vi "Find Missing Hardware Identifiers.vi"(8 "error in (no error)":errorcluster, 11 "Routing and Faulting Custom Device Ref in":T2 format="%.0x") -> (0 "error out":errorcluster, 1 "Identifier Errors":errorcluster[](array[cluster]), 2 "Missing Identifiers":T1[](array[typedef]), 3 "Routing and Faulting Custom Device Ref out":T2 format="%.0x")   [LabVIEW 2017, in "Routing and Faulting Scripting.lvlib"]
uses:
  Routing and Faulting Scripting.lvlib
  <vilib>/NI Veristand/Custom Device API/Custom Device Item Ref.ctl
  Identifier Path Pair.ctl
  NationalInstruments.VeriStand.SystemStorage
  Constants/Scripting Constants.vi
  <vilib>/NI Veristand/Custom Device API/Custom Device API.lvlib
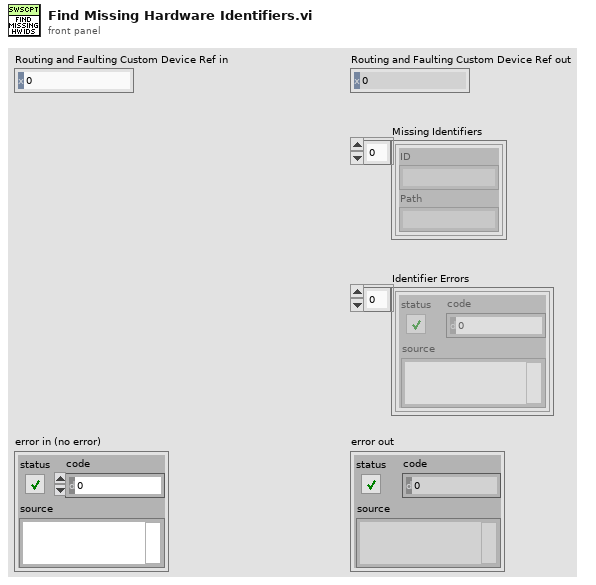
[diagram p1: front panel]
types:
  T1 = typedef "Routing and Faulting Scripting.lvlib/Identifier Path Pair.ctl" = cluster{"ID":string, "Path":string}
  T2 = typedef "Custom Device API.lvlib/Custom Device Item Ref.ctl" = u64
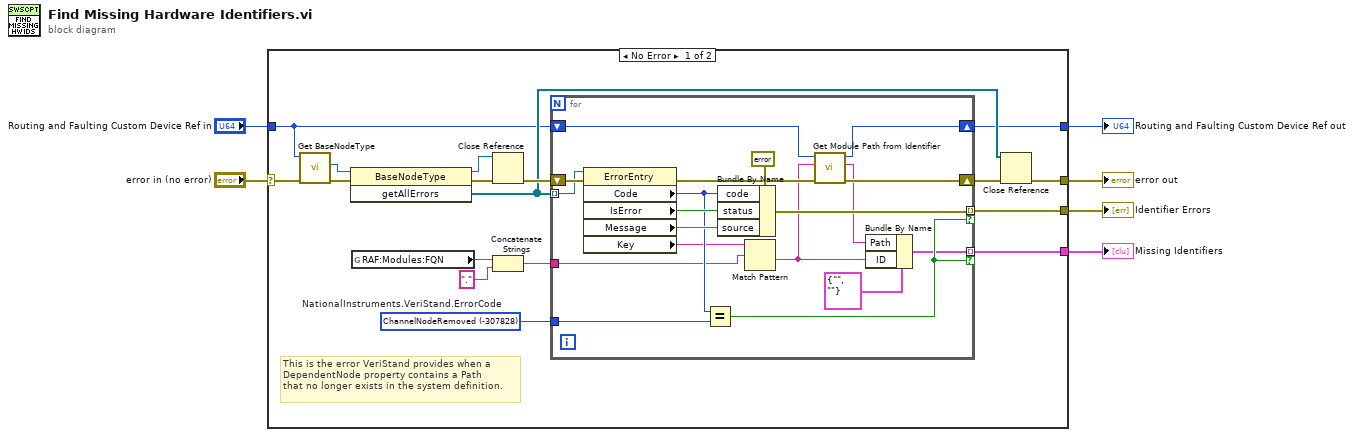
[diagram p0: block diagram]
diagram:
  n1 = case shown="No Error" "error in (no error)" {
    selector: "error in (no error)" -> [w15 w43]
    tunnel: "Routing and Faulting Custom Device Ref in" -> [w8 w44]
    tunnel: [w7 w44] -> w4
    tunnel: [w14 w43] -> w3
    tunnel: [w13 _] -> w2
    tunnel: [w12 _] -> w1
    frame No Error {
      w17 = -307828 items=["Success"=0, "NoProjectOpen"=-307992, "SequenceCompileError"=-307988, "SessionAlreadyDeployed"=-307984, "SessionNotDeployed"=-307982, "SequenceNotFoundInSession"=-307981, "StimulusProfileSessionLocked"=-307980, "EmptyNodeName"=-307930, "NodeAlreadyExistsByName"=-307926, "NumberOfCoefficientsOutOfRange"=-307884, "DownloadFileError"=-307872, "IncorrectLogFileName"=-307871, "LogTriggerConditionSyntaxError"=-307868, "DuplicateLogSessionName"=-307867, "LogSessionNotFound"=-307865, "ChannelLengthMismatch"=-307830, "NodeNotFoundDuringCompile"=-307829, "ChannelNodeRemoved"=-307828, "NotAChannel"=-307825, "NotAWaveform"=-307824, "STIFileError"=-307784, "DependenciesCycle"=-307783, "ChannelNotFoundInLogFile"=-307782, "ChannelGroupNotFoundInLogFile"=-307781, "GatewayNotOnLocalhost"=-307780, "NotEnoughDynamicDataSharingSpace"=-307738, "TargetMissingDataSharingDevice"=-307737, "ChannelMappingsSizeMismatch"=-307728, "DuplicateChannelAliasMappings"=-307711, "NotAnInlineCustomDevice"=-307710, "IncompatibleModel"=-307703, "ModelDimensionMismatch"=-307702, "SLSCChassisLoadFailed"=-307691, "TargetDisabled"=-307689, "MismatchedLengths"=-307687, "TargetInvalid"=-307686, "ParameterNotFound"=-307685, "ServerPortAlreadyInUse"=-307684, "TargetDisconnected"=-307682, "ServiceConfigurationFile"=-307681, "ModelParameterFileParseError"=-307680, "NoActionRequired"=-307677, "InputParameterInvalid"=-307676, "HostRunningDifferentSystemDefinition"=-307671, "ChannelNotScalable"=-307668, "ChannelCannotBeFaulted"=-307666, "ChannelNotWritable"=-307665, "ChannelNotReadable"=-307664, "Timeout"=-307663, "NodeNotFound"=-307662, "SystemDefinitionDeploymentFailure"=-307661, "SystemDefinitionDeploymentTimeout"=-307660, "EmptyPassword"=-307659, "SystemDefinitionAlreadyActive"=-307658, "InvalidConfigurationPassword"=-307657, "NoSystemDefinitionLoaded"=-307656, "ComponentNotAvailable"=-307655, "NotDeployed"=-307654, "InvalidFile"=-307653, "FailedServerConnection"=-307652, "FunctionNotSupported"=-307651, "UnexpectedError"=-307650, "UnmappedAlias"=-307617, "InvalidStreamConditionForDataType"=-307554, "WaveformDataTypeMismatch"=-307553, "InvalidDaqPluginFile"=-307526, "FileVersionUnsupported"=-307525]  # NationalInstruments.VeriStand.ErrorCode
      # "This is the error VeriStand provides when a\nDependentNode property contains a Path\nthat no longer exists in the system definition."
      n2 = call "Get BaseNodeType.vi"("error in (no error)"=w15, "Item Ref in"=w8) -> ("error out"=w23:errorcluster, "BaseNodeType"=w22:refnum<k24>)  [unwired: 7 in, 1 out]
      n3 = invoke class="BaseNodeType" method="getAllErrors"(reference=w22, error in=w23) -> (reference out=w20:refnum<k24>, error out=w21:errorcluster, "getAllErrors"=w16:refnum<k24>[])  [unwired: 1 in]
      n4 = global read "Scripting Constants.vi" "RAF:Modules:FQN"() -> (w11:string)
      n5 = Close Reference(reference=w20, error in (no error)=w21) -> (error out=w19:errorcluster)
      n6 = Concatenate Strings(w11, "." ("string")) -> (w9:string)
      n7 = for {
        shift-right: [w28] -> w18
        shift-left: w19 -> [w42]
        tunnel: w16 -> [w41] mode=indexing
        tunnel: [w37] -> w13 mode=indexing if=w34
        tunnel: w17 -> [w36]
        tunnel: [w24] -> w12 mode=indexing if=w34
        tunnel: w9 -> [w32]
        shift-right: [w29] -> w7
        shift-left: w8 -> [w30]
        n8 = property class="ErrorEntry"(reference=w41, error in=w42) -> (error out=w31:errorcluster, "Code"=w35:i32, "IsError"=w39:bool, "Message"=w38:string, "Key"=w33:string)  [unwired: 1 out]
        n9 = Equal?(x=w35, y=w36) -> (x = y?=w34:bool)
        n10 = Bundle By Name(cluster=errorcluster {"status"=FALSE, "code"=0, "source"=""} ("error out"), "code"=w35, "status"=w39, "source"=w38) -> (w37:errorcluster)
        n11 = Match Pattern(string=w33, regular expression=w32) -> (after substring=w26:string)  [unwired: 1 in, 3 out]
        n12 = call "Get Module Path from Identifier.vi"("error in (no error)"=w31, "Module identifier"=w26, "Routing and Faulting Ref in"=w30) -> ("error out"=w28:errorcluster, "Module path"=w25:string, "Routing and Faulting Ref out"=w29:T2)  [unwired: 6 in]
        n13 = Bundle By Name(cluster=T1 {"ID"="", "Path"=""}, "Path"=w25, "ID"=w26) -> (w24:T1)
      }
      n14 = Close Reference(reference=w16, error in (no error)=w18) -> (error out=w14:errorcluster)
    }
    frame Error {
    }
  }
  "Routing and Faulting Custom Device Ref out" <- w4
  "error out" <- w3
  "Identifier Errors" <- w2
  "Missing Identifiers" <- w1
